vi "Check Malfunction For A Sensor.vi"(1 "Mode":enum16{"Normally True", "Normally False"}(ring)=enum."Normally False", 2 "Logic Cluster":T1, 3 "Logic Status":bool, 4 "Current Pos":dbl) -> (0 "Malfunction?":bool)   [LabVIEW 2016, in "Hardware.lvlib" / "VacuumLine.lvlib" / "VacuumLine.lvclass"]
uses:
  <userlib>/Common Components/Hardware/Abstract System/VacuumLine/VacuumLine/VacuumLine.lvclass
  <userlib>/Common Components/Hardware/Abstract System/VacuumLine/VacuumLine/Logic Cluster.ctl
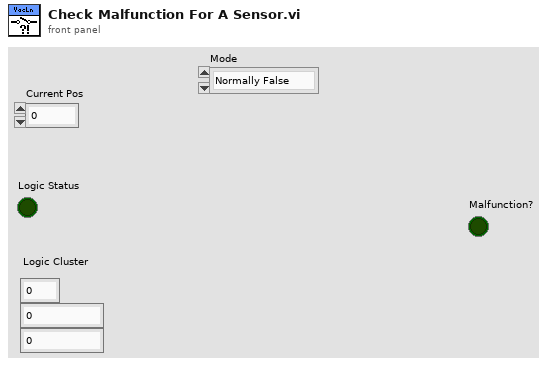
[diagram p1: front panel]
types:
  T1 = typedef "Hardware.lvlib/VacuumLine.lvlib/VacuumLine.lvclass/Logic Cluster.ctl" = cluster{"Pin#":u8, "Location":dbl, "Tolerance":dbl}
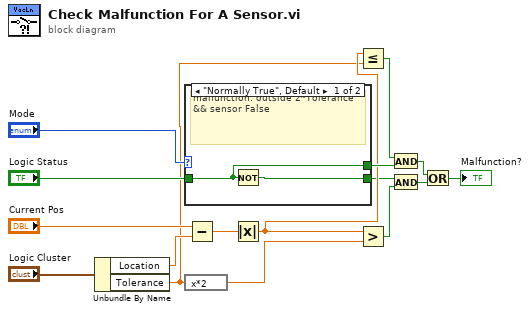
[diagram p0: block diagram]
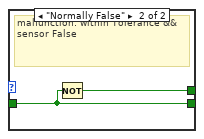
[diagram p2: hidden frame]
diagram:
  n1 = Unbundle By Name("Logic Cluster") -> ("Location"=w14:dbl, "Tolerance"=w6:dbl)
  n2 = case shown="\"Normally True\", Default" "Mode" {
    tunnel: "Logic Status" -> [w18 w19]
    tunnel: [w18 w20] -> w9
    tunnel: [w17 w19] -> w3
    frame "Normally True", Default {
      # "malfunction: outside 2*Tolerance && sensor False"
      n3 = Not(x=w18) -> (.not. x?=w17:bool)
    }
    frame "Normally False" {
      # "malfunction: within Tolerance && sensor False"
      n4 = Not(x=w19) -> (.not. x?=w20:bool)
    }
  }
  n5 = expression code="x*2"(w6) -> (w8:dbl)
  n6 = Subtract(x="Current Pos", y=w14) -> (x-y=w12:dbl)
  n7 = Absolute Value(x=w12) -> (abs(x)=w7:dbl)
  n8 = Less Or Equal?(x=w7, y=w6) -> (x <= y?=w5:bool)
  n9 = Greater?(x=w7, y=w8) -> (0:w4:bool)
  n10 = And(x=w5, y=w9) -> (x .and. y?=w10:bool)
  n11 = And(x=w3, y=w4) -> (x .and. y?=w1:bool)
  n12 = Or(x=w10, y=w1) -> (x .or. y?=→"Malfunction?":bool)
